vi "Ball Posession Status.vi"(7 "Override?":bool, 10 "Using Sensor?":bool, 11 "Sensor":bool) -> (3 "Ball Posessed?":bool)   [LabVIEW 2016]
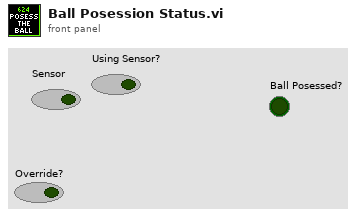
[diagram p1: front panel]
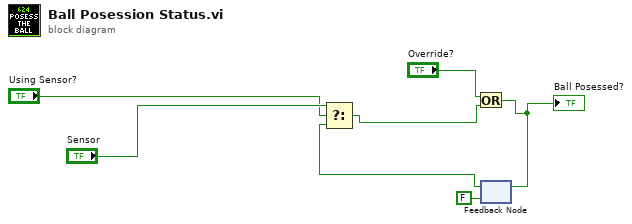
[diagram p0: block diagram]
diagram:
  n1 = feedback #1(FALSE ("Sensor")) -> (w3:bool)
  n2 = Select(t="Sensor", s="Using Sensor?", f=w3) -> (s? t:f=w1:bool)
  n3 = Or(x="Override?", y=w1) -> (x .or. y?=w6:bool)
  "Ball Posessed?" <- w6
  n4 = feedback-in #1(w6) -> ()
